vi "SR SIM921 Load Cal Curve.vi"(0 "VISA resource name":refnum<visa-resource-name>, 1 "Slot":T1(ring), 2 "Curve #":u32=1, 3 "Error In":errorcluster, 4 "Curve Data Format":T2(ring)=enum."LogLog") -> (5 "dup VISA resource name":refnum<visa-resource-name>, 6 "Error Out":errorcluster)   [LabVIEW 2020]
doc: "This VI will upload a calibration curve to the LakeShore 370 AC Resistance Bridge. It reads the data from a file and then formats it for uploading.\nScott Hannahs, <sth@magnet.fsu.edu> NHMFL-FSU, May 2003"
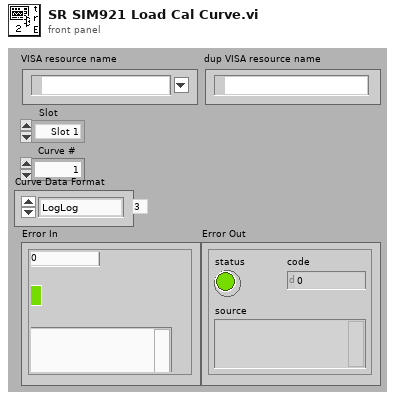
[diagram p1: front panel]
types:
  T1 = enum32{"Slot 1", "Slot 2", "Slot 3", "Slot 4", "Slot 5", "Slot 6", "Slot 7", "Slot 8"}
  T2 = enum16{"Linear", "SemiLogT", "SemiLogR", "LogLog"}
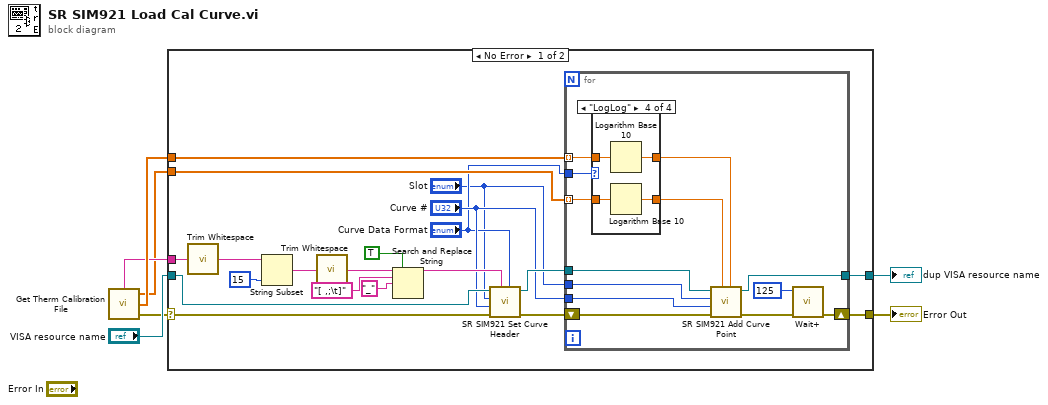
[diagram p0: block diagram]
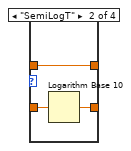
[diagram p3: hidden frame]
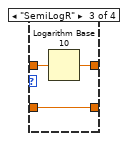
[diagram p4: hidden frame]
diagram:
  n1 = call "Get Therm Calibration File.vi"() -> ("Calbration Name"=w6:string, "Temperature"=w5:dbl[], "Resistance"=w7:dbl[], "error out"=w1:errorcluster)  [unwired: 1 in]
  n2 = case shown="No Error" w1 {
    selector: w1 -> [w18 w53]
    tunnel: w7 -> [w27 _]
    tunnel: w6 -> [w24 _]
    tunnel: w5 -> [w22 _]
    tunnel: "VISA resource name" -> [w21 w54]
    tunnel: [w20 w53] -> w3
    tunnel: [w19 w54] -> w2
    frame No Error {
      n3 = call <vilib>:"Trim Whitespace.vi"("string"=w24) -> ("trimmed string"=w14:string)  [unwired: 1 in]
      n4 = String Subset(string=w14, length (rest)=15 ("length (rest)")) -> (substring=w23:string)  [unwired: 1 in]
      n5 = call <vilib>:"Trim Whitespace.vi"("string"=w23) -> ("trimmed string"=w17:string)  [unwired: 1 in]
      n6 = Search and Replace String(replace all?=TRUE ("replace all? (F)"), input string=w17, search string="[ ,;\t]" ("replace string (\"\")"), replace string="_" ("replace string (\"\")")) -> (result string=w11:string)  [unwired: 4 in, 3 out]
      n7 = call "SR SIM921 Set Curve Header.vi"("Curve Data Format"="Curve Data Format", "Curve ID String"=w11, "Error In"=w18, "Curve #"="Curve #", "Slot"="Slot", "VISA resource name"=w21) -> ("Error Out"=w25:errorcluster, "VISA resource name"=w26:refnum<visa-resource-name>)  [unwired: 4 in]
      n8 = for {
        tunnel: w22 -> [w32] mode=indexing
        tunnel: w27 -> [w34] mode=indexing
        tunnel: w26 -> [w40]
        tunnel: "Curve #" -> [w30]
        tunnel: [w37] -> w19
        shift-right: [w36] -> w20
        shift-left: w25 -> [w39]
        tunnel: "Curve Data Format" -> [w33]
        tunnel: "Slot" -> [w31]
        n9 = case shown="\"LogLog\"" w33 {
          tunnel: w34 -> [w41 w43 w47 w49]
          tunnel: w32 -> [w42 w44 w48 w50]
          tunnel: [w41 w43 w46 w52] -> w28
          tunnel: [w42 w45 w48 w51] -> w29
          frame "Linear" {
          }
          frame "SemiLogT" {
            n10 = Logarithm Base 10(1:w44) -> (0:w45:dbl)
          }
          frame "SemiLogR" {
            n11 = Logarithm Base 10(1:w47) -> (0:w46:dbl)
          }
          frame "LogLog" {
            n12 = Logarithm Base 10(1:w49) -> (0:w52:dbl)
            n13 = Logarithm Base 10(1:w50) -> (0:w51:dbl)
          }
        }
        n14 = call "SR SIM921 Add Curve Point.vi"("Sensor"=w28, "Temperature"=w29, "Error In"=w39, "Curve #"=w30, "Slot"=w31, "VISA resource name"=w40) -> ("Error Out"=w38:errorcluster, "VISA resource name"=w37:refnum<visa-resource-name>)  [unwired: 4 in]
        n15 = call "Wait+.vi"("Error In"=w38, "milliseconds to wait"=u32 125) -> ("Error Out"=w36:errorcluster)  [unwired: 4 in, 1 out]
      }
    }
    frame Error {
    }
  }
  "Error Out" <- w3
  "dup VISA resource name" <- w2
